vi "Verify Errors.vi"(6 "This VI":refnum<vi>, 8 "STOP In":bool, 11 "error in":errorcluster) -> (0 "STOP Out":bool, 3 "error out":errorcluster)   [LabVIEW 2024, in "Error Handler.lvlib"]
uses:
  Error Handler.lvlib
  Support/General Type Defs/Error Handler Data.ctl
  Support/General Type Defs/Queue Message.ctl
  Error Queue - Enqueue.vi
  Support/General Type Defs/General Type Definitions.lvlib
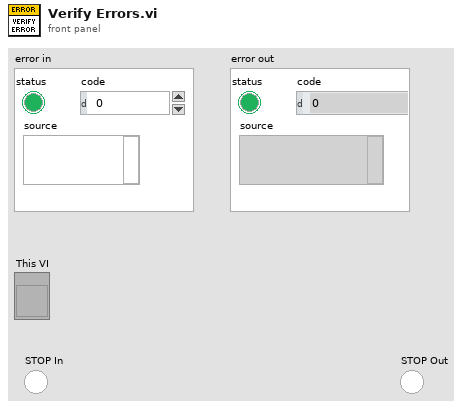
[diagram p1: front panel]
types:
  T1 = typedef "General Type Definitions.lvlib/Error Handler Data.ctl" = cluster{"Module":string, "Error Data":errorcluster, "Last Queue Message":T2}
  T2 = typedef "General Type Definitions.lvlib/Queue Message.ctl" = cluster{"Message":string, "Value":variant}
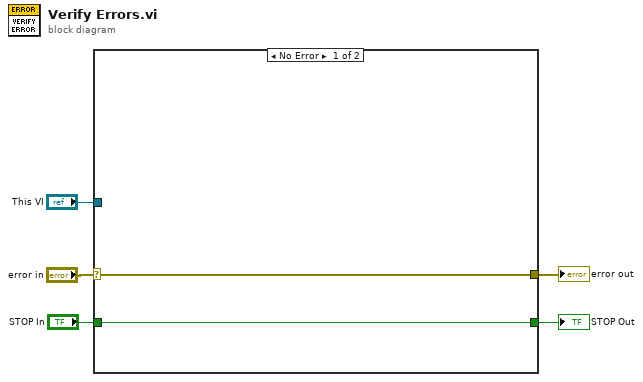
[diagram p0: block diagram]
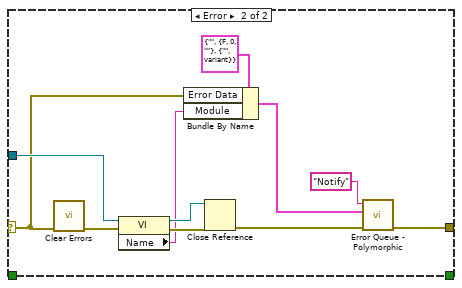
[diagram p2: hidden frame]
diagram:
  n1 = case shown="No Error" "error in" {
    selector: "error in" -> [w7 w9]
    tunnel: [w7 w15] -> w5
    tunnel: "This VI" -> [_ w12]
    tunnel: "STOP In" -> [w6 _]
    tunnel: [w6 _] -> w1
    frame No Error {
    }
    frame Error {
      n2 = call <vilib>:"Clear Errors.vi"("error in (no error)"=w9) -> ("error out"=w8:errorcluster)  [unwired: 5 in, 1 out]
      n3 = property class="VI"(reference=w12, error in=w8) -> (reference out=w13:refnum<vi>, error out=w14:errorcluster, "Name"=w11:string)
      n4 = Bundle By Name(cluster=T1 {"Module"="", "Error Data"={"status"=FALSE, "code"=0, "source"=""}, "Last Queue Message"={"Message"="", "Value"=variant}} ("Error Handler Data"), "Error Data"=w9, "Module"=w11) -> (w17:T1)
      n5 = Close Reference(reference=w13, error in (no error)=w14) -> (error out=w10:errorcluster)
      n6 = call-poly "Error Queue - Polymorphic.vi"("error in"=w10, "Value"=w17, "Message"="Notify") -> ("error out"=w15:errorcluster)  [unwired: 8 in]
    }
  }
  "error out" <- w5
  "STOP Out" <- w1
